vi "Measure MaxPStabilisation.vi"(4 "Sample Holder":dbl, 5 "Cell position":dbl, 6 "Scan Settings JV":T1={"Light intensity (Suns)"=1.0, "Pre-bias time (s)"=5.0, "Maximum voltage (V)"=0.0, "Minimum voltage (V)"=-1.4, "Range Options"=0, "1st scan FB to SC?"=TRUE, "Step Size (V)"=0.01, "Source Delay (s)"=0.01, "Inverted device"=FALSE, "Measure stabilized power output"=TRUE, "Stabilzation time (s)"=40.0, "Use Vmp from JV scan"=TRUE, "Stabization voltage (V)"=0.8, "Only stabilize best pixels"=TRUE, "Number of pixels to stabilize \nper substrate"=0, "Stabilization time step (s)"=1.0, "Use max power tracking"=FALSE, "Pre-bias voltage (V)"=-1.4, "No. of data point averages"=1.0, "No. of J-V averages"=1.0, "Integration time (ms)"=200.0} {"Number of pixels to stabilize \nper substrate" items=["1", "2", "3", "4", "5", "6", "7", "8"]; "Range Options" items=["Auto Range", "Semi-Auto Range", "100 uA", "1 mA", "10 mA", "100 mA", "1A"]}, 7 "Cell details cluster in":T2={"Measure?"=TRUE, "Area (cm^2)"=0.0, "Cell Label"="", "Cell Description"="", "Cell Position"=0, "Time in rig (s)"=0.0, "Time to next scan (s)"=0.0, "Scan number"=0.0, "When did you stick it in?"=0.0, "Time between scans (s)"=0.0, "Time of the last scan (s)"=0.0, "Scan settings in queue"=0, "Sample Holder"=0.0, "User Name"=""} {"Scan settings in queue" items=["Regular", "Inverted", "MartinaSettings"]; "Time of the last scan (s)" format="%<%H:%M:%S>t"; "When did you stick it in?" format="%<%H:%M:%S>t"; "Time to next scan (s)" format="%<%H:%M:%S>t"; "Time in rig (s)" format="%<%H:%M:%S>t"}, 8 "File path of master log":path, 10 "Experiment Title":string, 11 "User Name":string) -> (0 "Data Array":dbl[][](array[numeric]), 2 "Area (cm^2)":dbl, 3 "Jt Curve":cluster{"Y":dbl[], "Y":dbl[]}[](graph) caption="JV Curve")   [LabVIEW 2011]
uses:
  Typedefs/Queue cluster.ctl
  Typedefs/Scan settings.ctl
  <instrlib>/keithley_24xx/Keithley 24XX/Keithley 24XX.lvlib
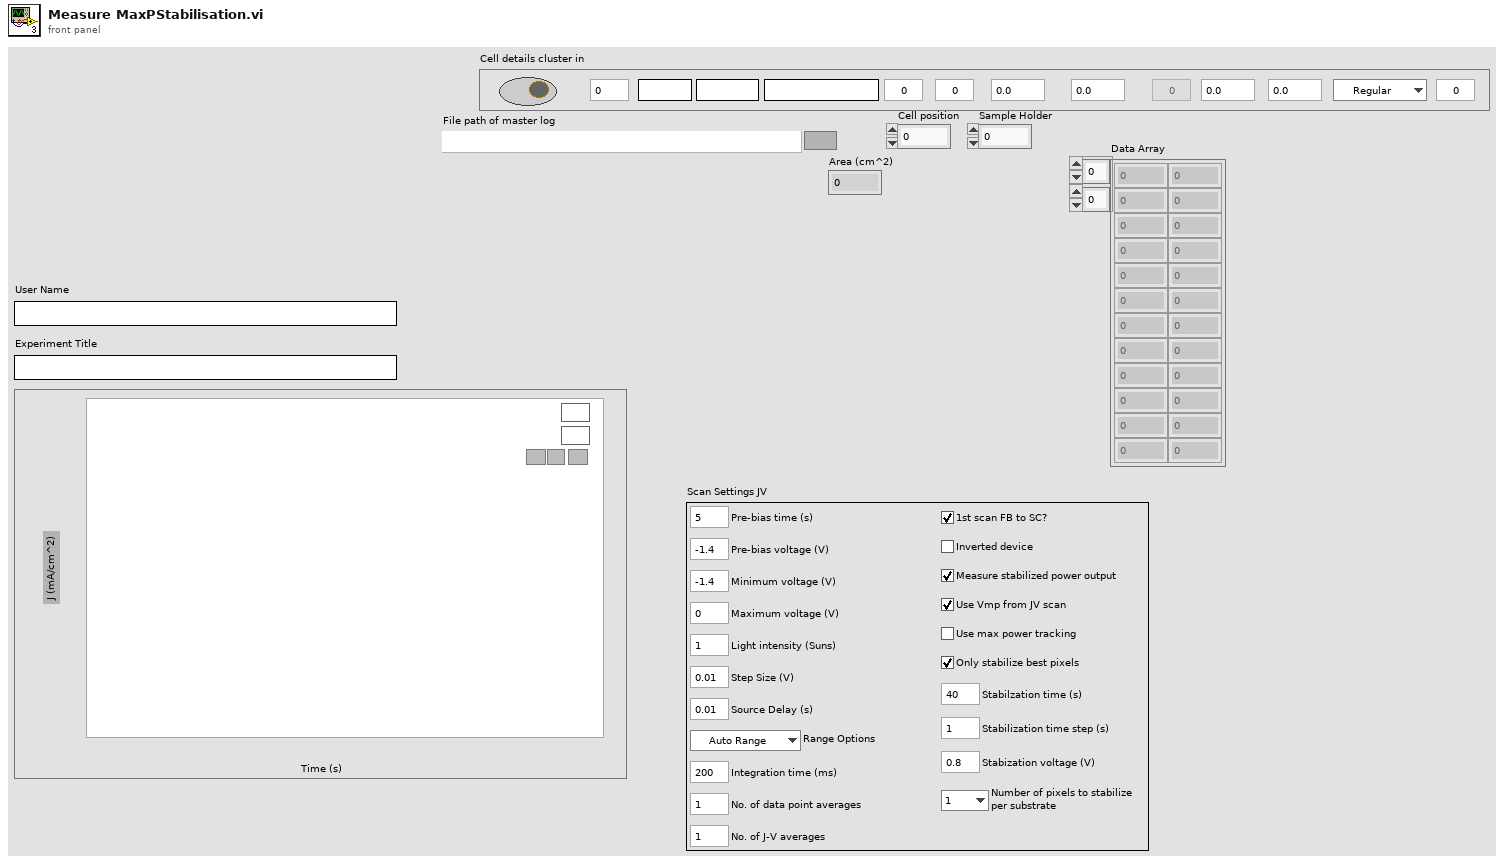
[diagram p1: front panel]
types:
  T1 = typedef "Scan settings.ctl" = cluster{"Light intensity (Suns)":dbl, "Pre-bias time (s)":dbl, "Maximum voltage (V)":dbl, "Minimum voltage (V)":dbl, "Range Options":u16, "1st scan FB to SC?":bool, "Step Size (V)":dbl, "Source Delay (s)":dbl, "Inverted device":bool, "Measure stabilized power output":bool, "Stabilzation time (s)":dbl, "Use Vmp from JV scan":bool, "Stabization voltage (V)":dbl, "Only stabilize best pixels":bool, "Number of pixels to stabilize \nper substrate":u16, "Stabilization time step (s)":dbl, "Use max power tracking":bool, "Pre-bias voltage (V)":dbl, "No. of data point averages":dbl, "No. of J-V averages":dbl, "Integration time (ms)":dbl}
  T2 = typedef "Queue cluster.ctl" = cluster{"Measure?":bool, "Area (cm^2)":dbl, "Cell Label":string, "Cell Description":string, "Cell Position":i32, "Time in rig (s)":dbl, "Time to next scan (s)":dbl, "Scan number":dbl, "When did you stick it in?":dbl, "Time between scans (s)":dbl, "Time of the last scan (s)":dbl, "Scan settings in queue":u16, "Sample Holder":dbl, "User Name":string}
  T3 = typedef "imagedata.ctl" = cluster{"image type":i32, "image depth":i32, "image":u8[], "mask":u8[], "colors":u32[], "Rectangle":cluster{"left":i16, "top":i16, "right":i16, "bottom":i16}}
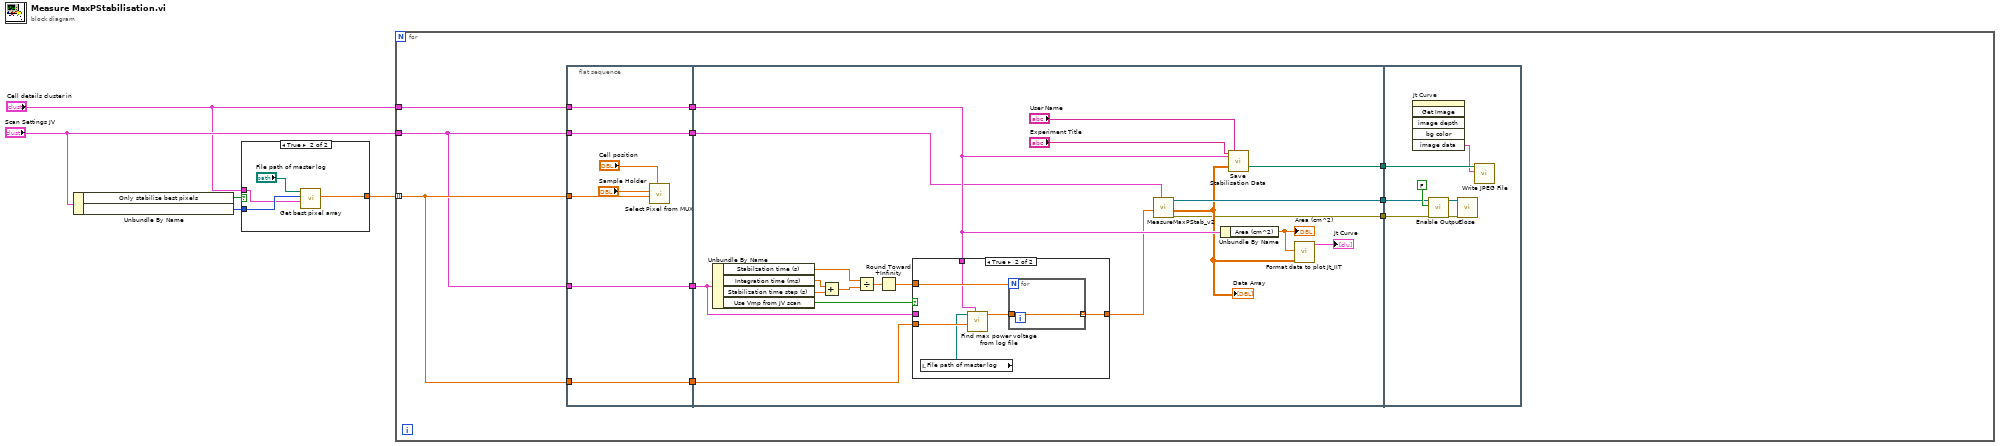
[diagram p0: block diagram]
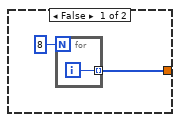
[diagram p2: hidden frame]
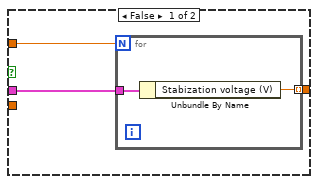
[diagram p3: hidden frame]
diagram:
  n1 = Unbundle By Name("Scan Settings JV") -> ("Only stabilize best pixels"=w5:bool, "Number of pixels to stabilize \nper substrate"=w3:u16)
  n2 = case shown="True" w5 {
    tunnel: [w6 w11] -> w4
    tunnel: w3 -> [_ w12]
    tunnel: "Cell details cluster in" -> [_ w10]
    frame False {
      n3 = for {
        N: 8 -> [_]
        tunnel: [w8] -> w6 mode=indexing
        i -> [w8]
      }
    }
    frame True {
      n4 = call "Get best pixel array.vi"("Cell details cluster"=w10, "Number of best pixels"=w12, "File path of master log"="File path of master log") -> ("Pixel Array"=w11:dbl[])  [unwired: 7 in, 1 out]
    }
  }
  n5 = for {
    tunnel: "Scan Settings JV" -> [w13]
    tunnel: w4 -> [w20] mode=indexing
    tunnel: "Cell details cluster in" -> [w15]
    n6 = flat-sequence {
      tunnel: w20 -> [w27]
      tunnel: w13 -> [w28]
      tunnel: w15 -> [w29]
      tunnel: [w29] -> w19
      tunnel: [w28] -> w18
      tunnel: [w27] -> w17
      tunnel: w20 -> [w26]
      tunnel: [w23] -> w14
      tunnel: w13 -> [w23]
      tunnel: [w48] -> w22
      tunnel: [w49] -> w21
      tunnel: w19 -> [w40]
      tunnel: w18 -> [w42]
      tunnel: w17 -> [w39]
      tunnel: [w36] -> w16
      tunnel: w14 -> [w34]
      tunnel: w22 -> [w63]
      tunnel: w21 -> [w65]
      tunnel: w16 -> [w62]
      frame #0 {
        n7 = call "Select Pixel from MUX.vi"("Cell position"="Cell position", "Pixel"=w26, "Sample Holder"="Sample Holder") -> ()  [unwired: 9 in]
      }
      frame #1 {
        n8 = Unbundle By Name(w42) -> ("Stabilzation time (s)"=w30:dbl, "Integration time (ms)"=w32:dbl, "Stabilization time step (s)"=w33:dbl, "Use Vmp from JV scan"=w41:bool)
        n9 = Add(x=w32, y=w33) -> (x+y=w31:dbl)
        n10 = Divide(x=w30, y=w31) -> (x/y=w44:dbl)
        n11 = Round Toward +Infinity(x=w44) -> (ceil(x): smallest int >= x=w43:dbl)
        n12 = case shown="True" w41 {
          tunnel: w43 -> [w52 w60]
          tunnel: w42 -> [w51 _]
          tunnel: [w50 w59] -> w38
          tunnel: w40 -> [_ w57]
          tunnel: w39 -> [_ w56]
          frame False {
            n13 = for {
              N: w52 -> [_]
              tunnel: w51 -> [w54]
              tunnel: [w53] -> w50 mode=indexing
              n14 = Unbundle By Name(w54) -> ("Stabization voltage (V)"=w53:dbl)
            }
          }
          frame True {
            n15 = local read "File path of master log"() -> (w55:path)
            n16 = call "Find max power voltage from log file.vi"("Cell details cluster in 2"=w57, "Pixel"=w56, "File path of master log"=w55) -> ("Vmp"=w58:dbl)  [unwired: 8 in]
            n17 = for {
              N: w60 -> [_]
              tunnel: [w61] -> w59 mode=indexing
              tunnel: w58 -> [w61]
            }
          }
        }
        n18 = call "MeasureMaxPStab_v2.vi"("Scan Settings JV"=w34, "Voltage List"=w38) -> ("error out"=w36:errorcluster, "Data Array"=w37:dbl[][], "VISA resource name out"=w48:refnum<visa-resource-name>)  [unwired: 7 in]
        "Data Array" <- w37
        n19 = Unbundle By Name(w40) -> ("Area (cm^2)"=w35:dbl)
        "Area (cm^2)" <- w35
        n20 = call "Save Stabilisation Data.vi"("Experiment Indicator"="Experiment Title", "Cell details cluster in"=w40, "Data Array"=w37, "Username"="User Name") -> ("File path for JV image"=w49:path)  [unwired: 14 in, 1 out]
        n21 = call "Format data to plot Jt_IIT.vi"("Data Array 2"=w37, "Device Area (cm^2)"=w35) -> ("JV Curve"=→"Jt Curve":cluster{"Y":dbl[], "Y":dbl[]}[])  [unwired: 9 in]
      }
      frame #2 {
        n22 = invoke on="Jt Curve" class="XYGraph (strict)" method="Get Image"() -> ("image data"=w64:T3)  [unwired: 6 in, 5 out]
        n23 = call <instrlib>:"Enable Output.vi"("error in (no error)"=w62, "Enable Output (T: Enable)"=FALSE ("Output (Off)"), "VISA resource name"=w63) -> ("error out"=w67:errorcluster, "VISA resource name out"=w68:refnum<visa-resource-name>)  [unwired: 7 in]
        n24 = call <instrlib>:"Close.vi"("error in (no error)"=w67, "VISA resource name"=w68) -> ()  [unwired: 9 in, 1 out]
        n25 = call <vilib>:"Write JPEG File.vi"("image data"=w64, "path to JPEG file"=w65) -> ()  [unwired: 8 in, 2 out]
      }
    }
  }
